vi "Get Local Chassis Slots Configuration.vi"(8 "error in (no error)":errorcluster, 11 "Item Ref in":T2 format="%.0x") -> (0 "error out":errorcluster, 2 "Slots Configuration":T1[](array[typedef]), 3 "Item Ref out":T2 format="%.0x")   [LabVIEW 2019, in "SEECD System Explorer.lvlib"]
doc: "This VI lists the module(s) configured in Local Chassis. GUIDs are used to create the list. The output is a list of Slot Number."
uses:
  SEECD System Explorer.lvlib
  <vilib>/NI VeriStand/Custom Device API/Custom Device Item Ref.ctl
  Type Defs/Slot Programming Mode.ctl
  Shared/Globals/Scan Engine GUIDs.vi
  <vilib>/NI VeriStand/Custom Device Tools/Custom Device Utility Library/NI VeriStand - Search for Item by GUID.vi
  Shared/Globals/Property Strings.vi
  <vilib>/NI VeriStand/Custom Device Tools/Custom Device Utility Library/Custom Device Utility Library.lvlib
  Shared/SEECD Shared.lvlib
  <vilib>/NI VeriStand/Custom Device API/Custom Device API.lvlib
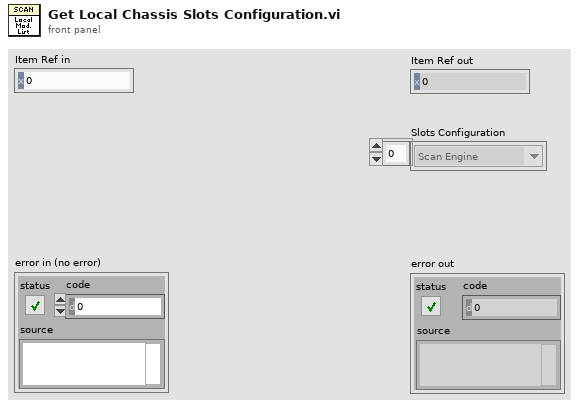
[diagram p1: front panel]
types:
  T1 = typedef "SEECD System Explorer.lvlib/Slot Programming Mode.ctl" = enum16{"Don't Modify", "Scan Engine", "LabVIEW FPGA", "NI-DAQmx"}
  T2 = typedef "Custom Device API.lvlib/Custom Device Item Ref.ctl" = u64
  T3 = typedef "Custom Device API.lvlib/Custom Device Item Info.ctl" = cluster{"Name":string, "Is Channel":bool, "GUID":string, "Is Waveform":bool}
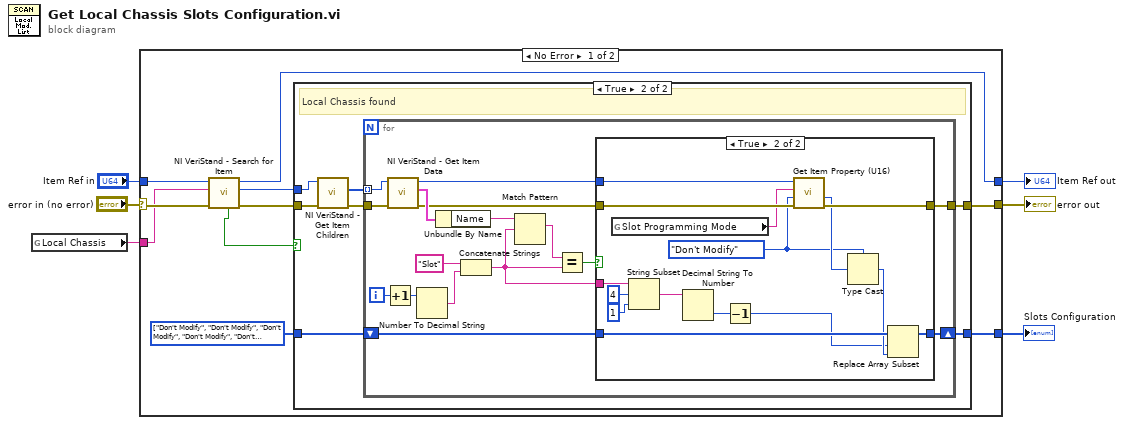
[diagram p0: block diagram]
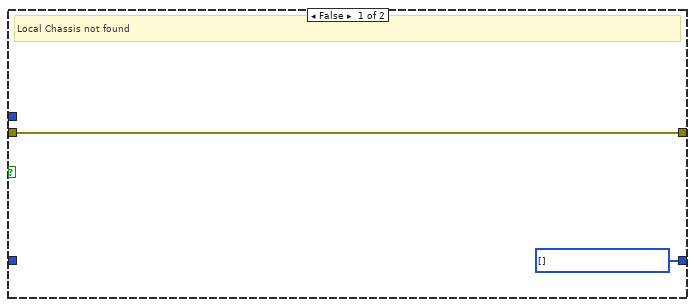
[diagram p2: hidden frame]
diagram:
  n1 = global read "Scan Engine GUIDs.vi" "Local Chassis"() -> (w3:string)
  n2 = case shown="No Error" "error in (no error)" {
    selector: "error in (no error)" -> [w16 w60]
    tunnel: [w9 w60] -> w5
    tunnel: "Item Ref in" -> [w15 w59]
    tunnel: w3 -> [w14 _]
    tunnel: [w10 w59] -> w2
    tunnel: [w8 _] -> w1
    frame No Error {
      w7 = T1[] [enum."Don't Modify", enum."Don't Modify", enum."Don't Modify", enum."Don't Modify", enum."Don't Modify", enum."Don't Modify", enum."Don't Modify", enum."Don't Modify"] items=["Don't Modify", "Scan Engine", "LabVIEW FPGA", "NI-DAQmx"] ("Slots Configuration")
      n3 = call-poly <vilib>:"NI VeriStand - Search for Item.vi"("error in"=w16, "Item GUID"=w14, "Section Ref in"=w15) -> ("error out"=w12:errorcluster, "Item Ref"=w11:T2, "Section Ref out"=w10:T2, "Found"=w13:bool)  [unwired: 5 in]
      n4 = case shown="True" w13 {
        tunnel: w12 -> [w18 w24]
        tunnel: w11 -> [_ w23]
        tunnel: [w18 w25] -> w9
        tunnel: [w17 w19] -> w8
        tunnel: w7 -> [_ w20]
        frame False {
          w17 = T1[] [] items=["Don't Modify", "Scan Engine", "LabVIEW FPGA", "NI-DAQmx"] ("Slots Configuration")
          # "Local Chassis not found"
        }
        frame True {
          # "Local Chassis found"
          n5 = call <vilib>:"NI VeriStand - Get Item Children.vi"("error in (no error)"=w24, "Item Ref in"=w23) -> ("error out"=w21:errorcluster, "Child Refs"=w22:T2[])  [unwired: 6 in, 2 out]
          n6 = for {
            tunnel: [w41] -> w25
            tunnel: w22 -> [w39] mode=indexing
            tunnel: w21 -> [w40]
            shift-right: [w27] -> w19
            shift-left: w20 -> [w28]
            i -> [w33]
            n7 = Increment(x=w33) -> (x+1=w32:i32)
            n8 = call <vilib>:"NI VeriStand - Get Item Data.vi"("error in (no error)"=w40, "Item Ref in"=w39) -> ("error out"=w37:errorcluster, "Item Info"=w38:T3, "Item Ref out"=w36:T2)  [unwired: 6 in, 1 out]
            n9 = Number To Decimal String(number=w32) -> (decimal integer string=w34:string)  [unwired: 1 in]
            n10 = Unbundle By Name(w38) -> ("Name"=w31:string)
            n11 = Concatenate Strings("Slot" ("string"), w34) -> (w26:string)
            n12 = Match Pattern(string=w31, regular expression=w26) -> (match substring=w30:string)  [unwired: 1 in, 3 out]
            n13 = Equal?(x=w30, y=w26) -> (x = y?=w29:bool)
            n14 = case shown="True" w29 {
              tunnel: w37 -> [w43 w58]
              tunnel: [w43 w57] -> w41
              tunnel: [w42 w47] -> w27
              tunnel: w36 -> [_ w53]
              tunnel: w28 -> [w42 w48]
              tunnel: w26 -> [_ w52]
              frame False {
              }
              frame True {
                w55 = Slot_Programming_Mode."Don't Modify" ("Slot Programming Mode 2")
                n15 = global read "Property Strings.vi" "Slot Programming Mode"() -> (w54:string)
                n16 = String Subset(string=w52, offset (0)=4, length (rest)=1 ("length (rest)")) -> (substring=w49:string)
                n17 = Decimal String To Number(string=w49) -> (number=w46:i32)  [unwired: 2 in, 1 out]
                n18 = Decrement(x=w46) -> (x-1=w44:i32)
                n19 = call <vilib>:"Get Item Property (U16).vi"("error in (no error)"=w58, "Default Value"=w55, "Property Name"=w54, "Item Ref in"=w53) -> ("error out"=w57:errorcluster, "Value"=w56:u16)  [unwired: 4 in, 2 out]
                n20 = Type Cast(type=w55, x=w56) -> (*(type *) &x=w45:T1)
                n21 = Replace Array Subset(array=w48, new element=w45, index=w44) -> (w47:T1[])
              }
            }
          }
        }
      }
    }
    frame Error {
    }
  }
  "Item Ref out" <- w2
  "error out" <- w5
  "Slots Configuration" <- w1
